vi "Direct_relay.vi"(10 "DOs":bool[](array[boolean]), 11 "Relay_Channel_Out":T1[](array[typedef])) -> (2 "Array":bool[](array[boolean]))   [LabVIEW 2024]
uses:
  Relay_Enum_OUT.ctl
  Relay_Channel_Write.ctl
  Relay_Module.lvlib
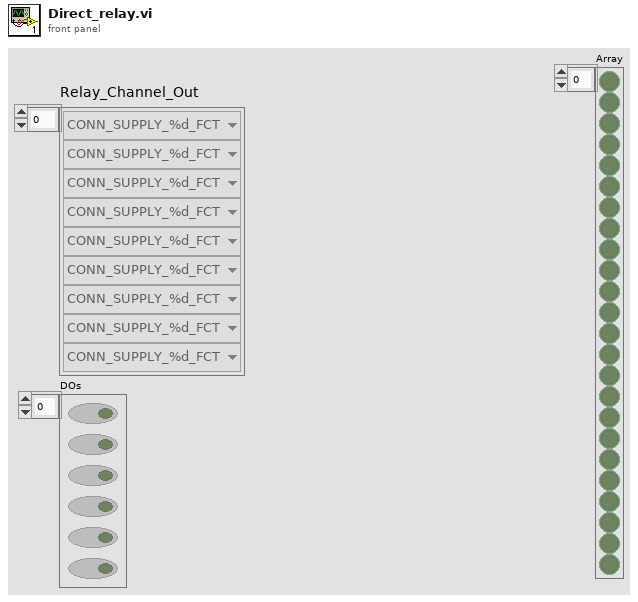
[diagram p1: front panel]
types:
  T1 = typedef "Relay_Module.lvlib/Relay_Enum_OUT.ctl" = enum16{"CONN_SUPPLY_%d_FCT", "HB_CONN_%d_FCT", "L_IND_CONN_%d_FCT", "R_IND_CONN_%d_FCT", "SW1_%d_FCT", "SW2_%d_FCT", "CAN_H_%d_FCT", "CAN_L_%d_FCT", "CYLINDER_ON/OFF_%d_FCT", "SPARE_1_%d_FCT", "SPARE_2_%d_FCT", "Tower Red", "Tower Amber", "Tower Green", "Tower Buzzer", "SLIMRELAY_DUT_%d_FCT", "GND_DMM_%d_EOL", "CAN_H_RES_%d_EOL", "CAN_L_RES_%d_EOL", "L_IND_RES_%d_EOL", "R_IND_RES_%d_EOL", "HB_CONN_DMM_%d_EOL", "14V_RES_%d_EOL", "CAN_L_(DMM-)_%d_EOL", "CAN_H_%d_EOL", "CAN_L_%d_EOL", "14V_%d_EOL", "GND_%d_EOL", "HB_CONN_%d_EOL", "L_IND_%d_EOL", "R_IND_%d_EOL", "CYLINDER_DUT_%d_EOL", "CYL_PB_1_%d_EOL", "CYL_PB_2_%d_EOL", "DUT_PASS_%d_EOL", "DUT_FAIL_%d_EOL", "SPARE1_%d_EOL", "Tower Red_EOL", "Tower Amber_EOL", "Tower Green_EOL", "Tower Buzzer_EOL"}
  T2 = typedef "Relay_Module.lvlib/Relay_Channel_Write.ctl" = cluster{"Relay_CH_Array":cluster{"On/Off":bool, "OUTPUT_Relay_Channels":T1}[]}
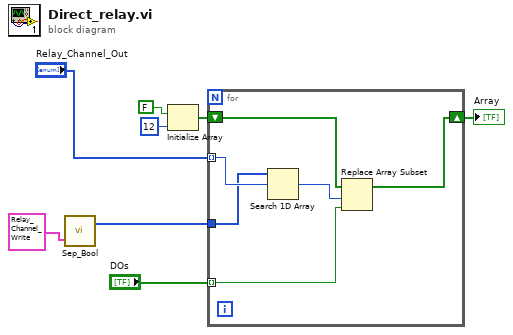
[diagram p0: block diagram]
diagram:
  n1 = call "Sep_Bool.vi"("output cluster"=T2 {"Relay_CH_Array"=[{"On/Off"=FALSE, "OUTPUT_Relay_Channels"=enum."CONN_SUPPLY_%d_FCT"}, {"On/Off"=FALSE, "OUTPUT_Relay_Channels"=enum."HB_CONN_%d_FCT"}, {"On/Off"=FALSE, "OUTPUT_Relay_Channels"=enum."L_IND_CONN_%d_FCT"}, {"On/Off"=FALSE, "OUTPUT_Relay_Channels"=enum."R_IND_CONN_%d_FCT"}, {"On/Off"=FALSE, "OUTPUT_Relay_Channels"=enum."SW1_%d_FCT"}, {"On/Off"=FALSE, "OUTPUT_Relay_Channels"=enum."SW2_%d_FCT"}, {"On/Off"=FALSE, "OUTPUT_Relay_Channels"=enum."CAN_H_%d_FCT"}, {"On/Off"=FALSE, "OUTPUT_Relay_Channels"=enum."CAN_L_%d_FCT"}, {"On/Off"=FALSE, "OUTPUT_Relay_Channels"=enum."CYLINDER_ON/OFF_%d_FCT"}, {"On/Off"=FALSE, "OUTPUT_Relay_Channels"=enum."SPARE_1_%d_FCT"}, {"On/Off"=FALSE, "OUTPUT_Relay_Channels"=enum."SPARE_2_%d_FCT"}, {"On/Off"=FALSE, "OUTPUT_Relay_Channels"=enum."Tower Red"}, {"On/Off"=FALSE, "OUTPUT_Relay_Channels"=enum."Tower Amber"}, {"On/Off"=FALSE, "OUTPUT_Relay_Channels"=enum."Tower Green"}, {"On/Off"=FALSE, "OUTPUT_Relay_Channels"=enum."Tower Buzzer"}, {"On/Off"=FALSE, "OUTPUT_Relay_Channels"=enum."SLIMRELAY_DUT_%d_FCT"}]} ("Relay_Channel_Write")) -> ("Array"=w6:T1[])  [unwired: 1 in, 1 out]
  n2 = Initialize Array(FALSE, 12 ("dimension size")) -> (w2:bool[])
  n3 = for {
    tunnel: "Relay_Channel_Out" -> [w14] mode=indexing
    tunnel: w6 -> [w13]
    tunnel: "DOs" -> [w11] mode=indexing
    shift-right: [w9] -> w1
    shift-left: w2 -> [w10]
    n4 = Search 1D Array(1D array=w13, element=w14) -> (index of element=w12:i32)  [unwired: 1 in]
    n5 = Replace Array Subset(array=w10, new element=w11, index=w12) -> (w9:bool[])
  }
  "Array" <- w1
